vi "Execute.Initialize.vi"(8 "error in (no error)":errorcluster, 11 "Cluster":T1={"NIVS.BaseLogPath"=path "", "NIVS.SystemDefinitionFile"=path "", "NIVS.Events"={"SequenceEvent"=refnum, "SystemChangeEvent"=refnum, "WorkspaceEvent"=refnum}, "NIVS.SequenceState"=enum."Idle", "NIVS.GatewayIPAddress"="", "NIVS.DataLogSpecRef"=refnum, "NIVS.DataLogManagerRef"=refnum, "NIVS.LogSessionGUID"="", "NIVS.WorkspaceManager"=refnum, "NIVS.Deployed"=FALSE, "NIVS.ProfileRef"=refnum, "NIVS.ProfileCallback"=refnum, "NIVS.SystemStateRefs"={"CustDatRef"=refnum, "EvtRef"=refnum, "Target State User Event"=refnum}, "UI.Abort"=refnum, "UI.Pause"=refnum, "UI.EnableLogging"=refnum, "UI.Start"=refnum, "UI.LogChannels"=refnum, "UI.StartIteration"=refnum, "UI.StartStep"=refnum, "UI.Sequence"=refnum, "UI.PreviewMode"=refnum, "UI.Graph"=refnum, "UI.BaseFileName"=refnum, "UI.Profiles"=refnum, "UI.CurrentStep"=refnum, "UI.CurrentIteration"=refnum, "UI.TotalIterations"=refnum, "Sequence.AbortChannel"="", "Sequence.StepInfoChannel"="", "Sequence.Iterations"=0, "Sequence.IterationInfoChannel"="", "Sequence.#ofColumns"=0, "Events.State"=refnum, "Events.Test Result"=refnum, "Events.Progress"=refnum, "INI.Settings"={"Build Location"=path "C:/Simple Sequence Editor/SequenceRepo", "LoggingLocation"=path ""}, "UI.Skip"=refnum, "Sequence.SkipChannel"="", "Restart.Path"=path "", "UI.Duration"=refnum, "Sequence.DurationChannel"=""}) -> (0 "error out":errorcluster)   [LabVIEW 2015, in "Simple Sequence Tools - Execution.lvlib"]
uses:
  Simple Sequence Tools - Execution.lvlib
  Types/Main.StateVariables.ctl
  Types/Execute.UserEventRefs.ctl
  <vilib>/NI Veristand/Execution/Workspace/SystemStateRegEventRef.ctl
  <vilib>/NI Veristand/Execution/Workspace/Target State Info.ctl
  <vilib>/NI Veristand/Execution/Workspace/Target State.ctl
  Types/Execution.SequenceState.ctl
  <vilib>/NI Veristand/Execution/DataLogging/DataLoggingSpecification Ref.ctl
  NationalInstruments.VeriStand.ClientAPI
  <vilib>/NI Veristand/Execution/DataLogging/IDataLogging Ref.ctl
  <vilib>/NI Veristand/Execution/Workspace/WorkspaceAPI.ctl
  NationalInstruments.VeriStand.RealTimeSequenceDefinitionApi
  <vilib>/NI Veristand/Execution/Workspace/SystemStateEventRef.ctl
  Shared/Types/INI.Settings
  Types/Execute.PreviewMode.ctl
  Shared/SubVIs/Main.Constants.vi
  Shared/Simple Sequence Tools - Shared.lvlib
  <vilib>/NI Veristand/Execution/Workspace/NI_VS Workspace ExecutionAPI.lvlib
  <vilib>/NI Veristand/Execution/DataLogging/NI_VS Data Logging API.lvlib
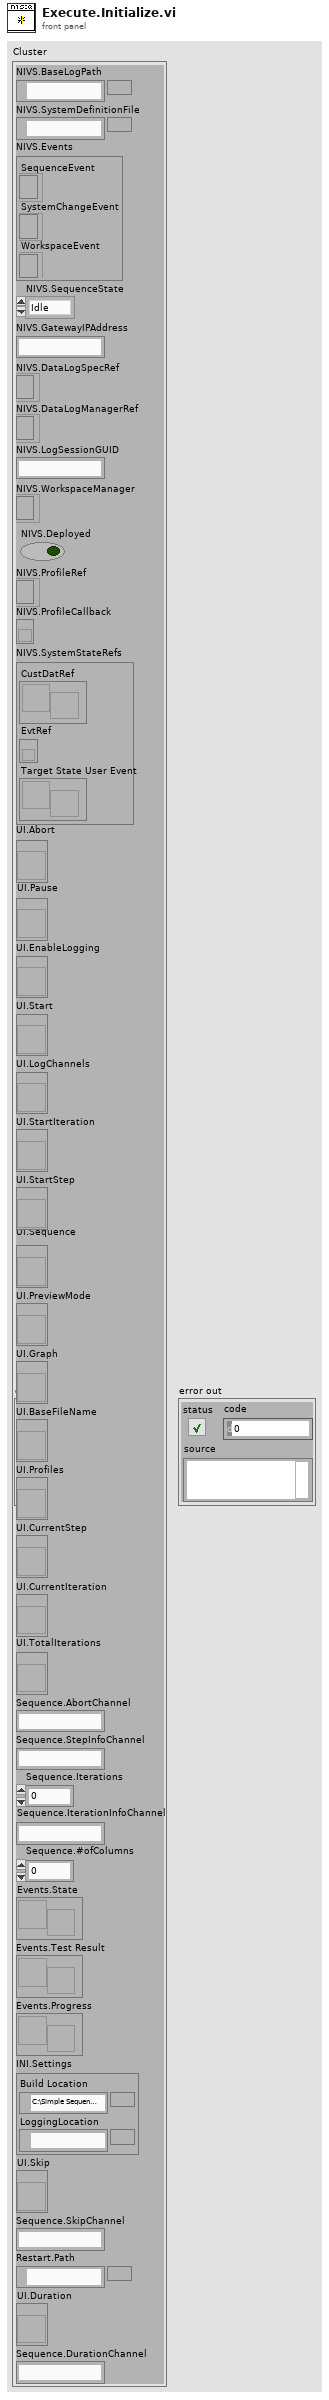
[diagram p1: front panel]
types:
  T1 = typedef "Simple Sequence Tools - Execution.lvlib/Main.StateVariables.ctl" = cluster{"NIVS.BaseLogPath":path, "NIVS.SystemDefinitionFile":path, "NIVS.Events":T2, "NIVS.SequenceState":T4, "NIVS.GatewayIPAddress":string, "NIVS.DataLogSpecRef":T5, "NIVS.DataLogManagerRef":T6, "NIVS.LogSessionGUID":string, "NIVS.WorkspaceManager":T7, "NIVS.Deployed":bool, "NIVS.ProfileRef":refnum<k24>, "NIVS.ProfileCallback":refnum<k27>, "NIVS.SystemStateRefs":T8, "UI.Abort":refnum<vi>, "UI.Pause":refnum<vi>, "UI.EnableLogging":refnum<vi>, "UI.Start":refnum<vi>, "UI.LogChannels":refnum<vi>, "UI.StartIteration":refnum<vi>, "UI.StartStep":refnum<vi>, "UI.Sequence":refnum<vi>, "UI.PreviewMode":refnum<vi>, "UI.Graph":refnum<vi>, "UI.BaseFileName":refnum<vi>, "UI.Profiles":refnum<vi>, "UI.CurrentStep":refnum<vi>, "UI.CurrentIteration":refnum<vi>, "UI.TotalIterations":refnum<vi>, "Sequence.AbortChannel":string, "Sequence.StepInfoChannel":string, "Sequence.Iterations":u32, "Sequence.IterationInfoChannel":string, "Sequence.#ofColumns":i32, "Events.State":refnum<user-event>, "Events.Test Result":refnum<user-event>, "Events.Progress":refnum<user-event>, "INI.Settings":T9, "UI.Skip":refnum<vi>, "Sequence.SkipChannel":string, "Restart.Path":path, "UI.Duration":refnum<vi>, "Sequence.DurationChannel":string}
  T2 = typedef "Simple Sequence Tools - Execution.lvlib/Execute.UserEventRefs.ctl" = cluster{"SequenceEvent":refnum<event-registration>, "SystemChangeEvent":T3, "WorkspaceEvent":refnum<event-registration>}
  T3 = typedef "NI_VS Workspace ExecutionAPI.lvlib/SystemStateRegEventRef.ctl" = refnum<event-registration>
  T4 = typedef "Simple Sequence Tools - Execution.lvlib/Execution.SequenceState.ctl" = enum16{"Idle", "Initializing", "Running", "Paused", "Finalizing", "Complete"}
  T5 = typedef "NI_VS Data Logging API.lvlib/DataLoggingSpecification Ref.ctl" = refnum<k24>
  T6 = typedef "NI_VS Data Logging API.lvlib/IDataLogging Ref.ctl" = refnum<k24>
  T7 = typedef "NI_VS Workspace ExecutionAPI.lvlib/WorkspaceAPI.ctl" = refnum<k24>
  T8 = typedef "NI_VS Workspace ExecutionAPI.lvlib/SystemStateEventRef.ctl" = cluster{"CustDatRef":refnum<user-event>, "EvtRef":refnum<k27>, "Target State User Event":refnum<user-event>}
  T9 = typedef "Simple Sequence Tools - Shared.lvlib/INI.Settings" = cluster{"Build Location":path, "LoggingLocation":path}
  T10 = enum8{"Enabled", "Disabled", "Disabled and Grayed Out"}
  T11 = typedef "Simple Sequence Tools - Execution.lvlib/Execute.PreviewMode.ctl" = enum8{"Graph", "Table"}
  T12 = enum16{"Channels (No System Channel)", "Aliases", "All"}
  T13 = typedef "LVBoundsTypeDef.ctl" = cluster{"Width":u32, "Height":u32}
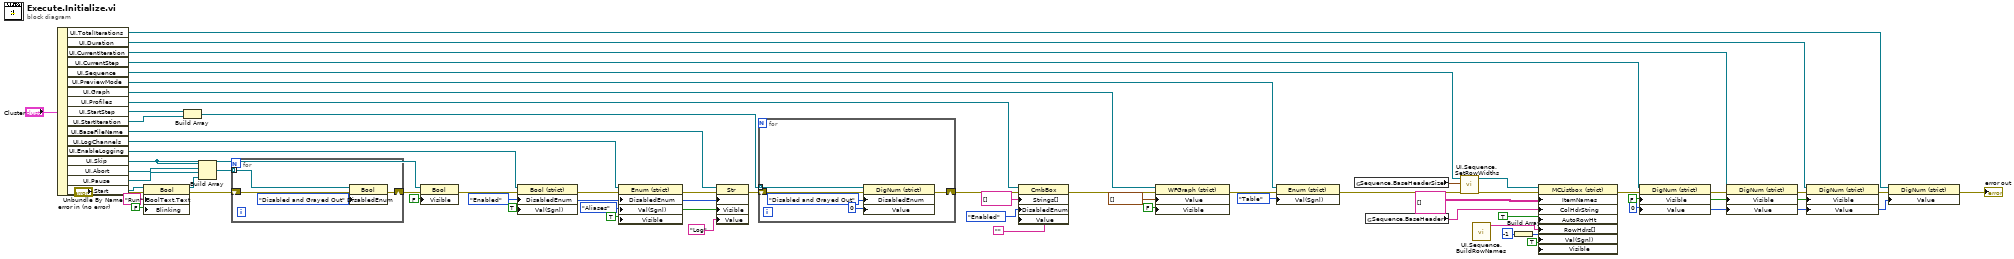
[diagram p0: block diagram]
diagram:
  w1 = u32 0 ("Value")
  w2 = FALSE ("Visible")
  w25 = TRUE ("Visible")
  w28 = T10."Enabled" ("Disabled")
  n1 = Unbundle By Name("Cluster") -> ("UI.TotalIterations"=w18:refnum<vi>, "UI.Duration"=w3:refnum<vi>, "UI.CurrentIteration"=w22:refnum<vi>, "UI.CurrentStep"=w23:refnum<vi>, "UI.Sequence"=w63:refnum<vi>, "UI.PreviewMode"=w51:refnum<vi>, "UI.Graph"=w48:refnum<vi>, "UI.Profiles"=w45:refnum<vi>, "UI.StartStep"=w42:refnum<vi>, "UI.StartIteration"=w41:refnum<vi>, "UI.BaseFileName"=w29:refnum<vi>, "UI.LogChannels"=w38:refnum<vi>, "UI.EnableLogging"=w37:refnum<vi>, "UI.Skip"=w13:refnum<vi>, "UI.Abort"=w34:refnum<vi>, "UI.Pause"=w35:refnum<vi>, "UI.Start"=w7:refnum<vi>)
  n2 = property class="Bool"(reference=w7, error in="error in (no error)", "BoolText.Text"="Run" ("Boolean Text.Text"), "Blinking"=FALSE) -> (reference out=w6:refnum<vi>, error out=w10:errorcluster)
  n3 = Build Array(w42, w41) -> (w43:refnum<vi>[])
  n4 = Build Array(w13, w34, w35, w6) -> (w36:refnum<vi>[])
  n5 = for {
    tunnel: w36 -> [w67] mode=indexing
    shift-right: [w65] -> w15
    shift-left: w10 -> [w64]
    n6 = property class="Bool"(reference=w67, error in=w64, "DisabledEnum"=T10."Disabled and Grayed Out" ("Disabled")) -> (error out=w65:errorcluster)  [unwired: 1 out]
  }
  n7 = property class="Bool"(reference=w13, error in=w15, "Visible"=FALSE) -> (error out=w14:errorcluster)  [unwired: 1 out]
  n8 = property class="Bool (strict)"(reference=w37, error in=w14, "DisabledEnum"=w28, "Val(Sgnl)"=TRUE ("Value (Signaling)")) -> (error out=w39:errorcluster)  [unwired: 1 out]
  n9 = property class="Enum (strict)"(reference=w38, error in=w39, "DisabledEnum"=w28, "Val(Sgnl)"=T12."Aliases" ("Value (Signaling)"), "Visible"=w25) -> (error out=w27:errorcluster)  [unwired: 1 out]
  n10 = property class="Str"(reference=w29, error in=w27, "DisabledEnum"=w28, "Visible"=w25, "Value"="Log") -> (error out=w26:errorcluster)  [unwired: 1 out]
  n11 = for {
    tunnel: w43 -> [w72] mode=indexing
    shift-right: [w70] -> w44
    shift-left: w26 -> [w69]
    n12 = property class="DigNum (strict)"(reference=w72, error in=w69, "DisabledEnum"=T10."Disabled and Grayed Out" ("Disabled"), "Value"=u32 0) -> (error out=w70:errorcluster)  [unwired: 1 out]
  }
  n13 = property class="CmbBox"(reference=w45, error in=w44, "Strings[]"=string[] [] ("Strings []"), "DisabledEnum"=T10."Enabled" ("Disabled"), "Value"="") -> (error out=w47:errorcluster)  [unwired: 1 out]
  n14 = property class="WFGraph (strict)"(reference=w48, error in=w47, "Value"=waveform(dbl)[] [], "Visible"=FALSE) -> (error out=w52:errorcluster)  [unwired: 1 out]
  n15 = property class="Enum (strict)"(reference=w51, error in=w52, "Val(Sgnl)"=Execute.PreviewMode."Table" ("View")) -> (error out=w62:errorcluster)  [unwired: 1 out]
  n16 = global read "Main.Constants.vi" "Sequence.BaseHeaderSize"() -> (w57:T13[])
  n17 = global read "Main.Constants.vi" "Sequence.BaseHeader"() -> (w56:string[])
  n18 = call "UI.Sequence.SetRowWidths.vi"("error in (no error)"=w62, "CellSize"=w57, "UI.SequenceRef"=w63) -> ("error out"=w61:errorcluster, "UI.SequenceRef"=w54:refnum<vi>)  [unwired: 7 in]
  n19 = call "UI.Sequence.BuildRowNames.vi"() -> ("Row Headings"=w59:string[])  [unwired: 11 in]
  n20 = Build Array(-1 ("Value")) -> (w58:i32[])
  n21 = property class="MCListbox (strict)"(reference=w54, error in=w61, "ItemNames"=string[][] [] ("Item Names"), "ColHdrString"=w56, "AutoRowHt"=TRUE ("Autosizing Row Height"), "RowHdrs[]"=w59, "Val(Sgnl)"=w58, "Visible"=TRUE) -> (error out=w20:errorcluster)  [unwired: 1 out]
  n22 = property class="DigNum (strict)"(reference=w23, error in=w20, "Visible"=w2, "Value"=w1) -> (error out=w21:errorcluster)  [unwired: 1 out]
  n23 = property class="DigNum (strict)"(reference=w22, error in=w21, "Visible"=w2, "Value"=w1) -> (error out=w5:errorcluster)  [unwired: 1 out]
  n24 = property class="DigNum (strict)"(reference=w3, error in=w5, "Visible"=w2, "Value"=w1) -> (error out=w4:errorcluster)  [unwired: 1 out]
  n25 = property class="DigNum (strict)"(reference=w18, error in=w4, "Value"=w1) -> (error out=→"error out":errorcluster)  [unwired: 1 out]
